vi "U8布尔之间转换.vi"() -> ()   [LabVIEW 2011]
panel:
  out "布尔类型转换回U8类型":u8
  out "U8类型转换成布尔类型":bool
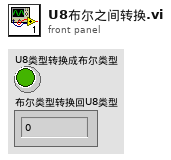
[diagram p1: front panel]
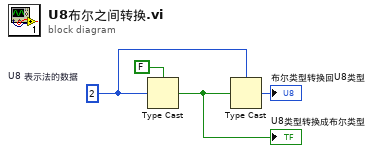
[diagram p0: block diagram]
diagram:
  w3 = u8 2  # U8 表示法的数据
  n1 = Type Cast(type=FALSE, x=w3) -> (*(type *) &x=w2:bool)
  "U8类型转换成布尔类型" <- w2
  n2 = Type Cast(type=w3, x=w2) -> (*(type *) &x=→"布尔类型转换回U8类型":u8)
